vi "Rising Edge.vi"(1 "Signal":bool) -> (0 "Rising Edge":bool)   [LabVIEW 2017, in "CSM Shared.lvlib"]
uses:
  CSM Shared.lvlib
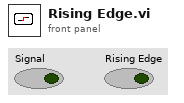
[diagram p1: front panel]
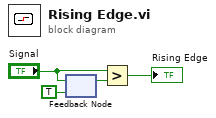
[diagram p0: block diagram]
diagram:
  n1 = feedback #1(TRUE) -> (w1:bool)
  n2 = feedback-in #1("Signal") -> ()
  n3 = Greater?(x="Signal", y=w1) -> (0:→"Rising Edge":bool)
